vi "TcpProtocoalUnderstandingClientSideServer.vi"() -> ()   [LabVIEW 2019]
panel:
  in  "stop":bool
  in  "Thermometer":dbl(slide) scale=0.0..100.0
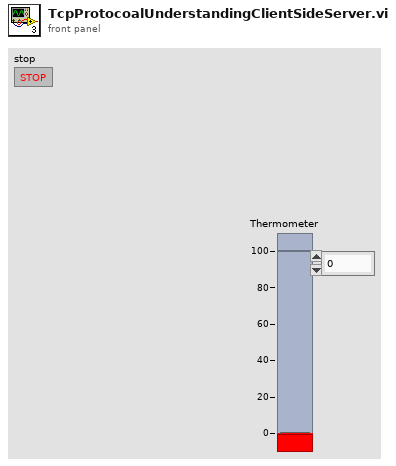
[diagram p1: front panel]
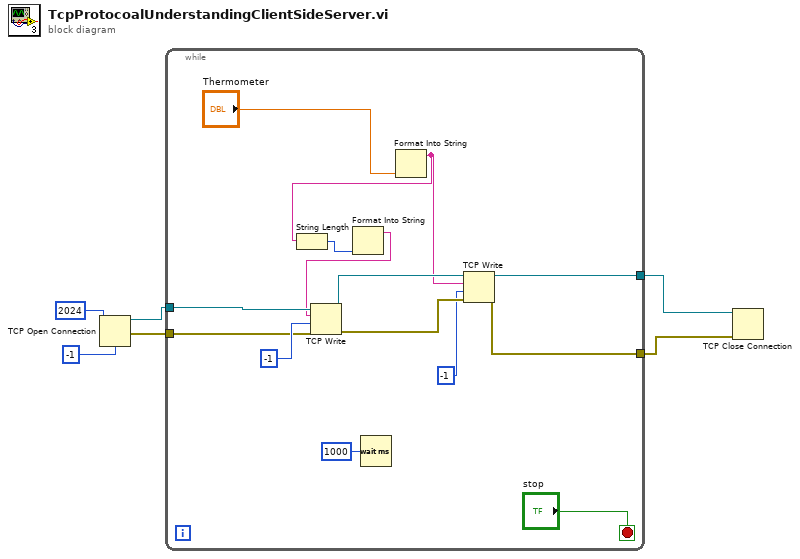
[diagram p0: block diagram]
diagram:
  n1 = TCP Open Connection(remote port or service name=u16 2024, timeout ms (60000)=-1) -> (connection ID=w1:refnum<k5>, error out=w2:errorcluster)  [unwired: 3 in]
  n2 = while {
    tunnel: [w19] -> w6
    tunnel: [w17] -> w5
    tunnel: w2 -> [w13]
    tunnel: w1 -> [w12]
    stop <- "stop" stop-if-true
    n3 = Wait (ms)(milliseconds to wait=u32 1000) -> ()  [unwired: 1 out]
    n4 = Format Into String "Format Into String"("Thermometer") -> (resulting string=w9:string)  [unwired: 3 in, 1 out]
    n5 = String Length(string=w9) -> (length=w10:i32)
    n6 = Format Into String(w10) -> (resulting string=w8:string)  [unwired: 3 in, 1 out]
    n7 = TCP Write(connection ID=w12, data in=w8, error in (no error)=w13, 9:-1 ("timeout ms (25000)")) -> (connection ID out=w20:refnum<k5>, error out=w18:errorcluster)  [unwired: 1 out]
    n8 = TCP Write(connection ID=w20, data in=w9, error in (no error)=w18, 9:-1 ("timeout ms (25000)")) -> (connection ID out=w19:refnum<k5>, error out=w17:errorcluster)  [unwired: 1 out]
  }
  n9 = TCP Close Connection(connection ID=w6, error in (no error)=w5) -> ()  [unwired: 1 in, 2 out]
